vi "cRIO9159_DAQDMA.vi"() -> ()   [LabVIEW 2013]
uses:
  datatypes/statesdaq.ctl
  <vilib>/rvi/Emulation/niFpgaSctlEmulationGetInTimedLoop.vi
  <vilib>/rvi/Emulation/niFpgaEmulationReportErrorSimple.vi
  <vilib>/rvi/Emulation/niFpgaGetClockAttributes.vi
  <vilib>/rvi/eio/common/nirviEmuTemplatePropertyGet_noerrors.vi
  <vilib>/rvi/eio/common/nirviEmuTemplateMethod_errors.vi
  <vilib>/rvi/Emulation/niFpgaCriticalErrorInLSC.vi
  <vilib>/rvi/interface/RandomDataEmulation/nirviRandomDataFPGAFIFO.vi
  <vilib>/rvi/interface/RandomDataEmulation/niFpgaRandomDataHandleErrors.vi
  <vilib>/eio/EIOPropertyNode/EIOPropertyNode.xnode
  <vilib>/eio/EIOMethodNode/EIOMethodNode.xnode
  <vilib>/eio/EIONode/EIONode.xnode
  <vilib>/rvi/DataTransferAndStorage/Container/XNode/niFpgaContainer.xnode
  <vilib>/rvi/interface/RandomDataEmulation/nirviRandomDataFpgaReadWriteTemplate.vi
  <vilib>/rvi/eio/common/nirviEmuTemplatePropertyGet_errors.vi
  <vilib>/rvi/eio/common/nirviEmuTemplatePropertySet_errors.vi
  <vilib>/rvi/eio/common/nirviEmuTemplatePropertySet_noerrors.vi
panel:
  in  "Loop(uSec)":u32=1000 caption="Count(uSec)"
  in  "Tab Control":T1(tab)=enum."Mandatory Resources"
  out "Platform":enum8{"FlexRIO", "cRIO", "RSeries"}(ring)=enum."cRIO"
  out "FPGAVIversion":u8[](array[numeric])=[1, 1]
  out "InitDone":bool
  out "Fref":u32=1000
  out "DevQualityStatus":u8
  out "DevTemp":i16=-9378
  out "DevProfile":u8
  in  "DAQStartStop":bool
  in  "DebugMode":bool
  out "InsertedIOModulesID":u16[](array[numeric])
  out "cRIOModulesOK":bool
  out "DMATtoHOSTBlockNWords":u16[](array[numeric])=[128]
  out "DMATtoHOSTNCh":u16[](array[numeric])=[2]
  out "DMATtoHOSTFrameType":u8[](array[numeric])
  out "DMATtoHOSTSampleSize":u8[](array[numeric])=[4]
  out "DMATtoHOSTOverflows":u16
  in  "DMATtoHOSTSamplingRate0":u16=1
  in  "DMATtoHOSTEnable0":bool
  out "SGFref0":u32=10000
  in  "AOEnable2":bool
  in  "AOEnable1":bool
  out "SGNo":u8=1
  in  "AO0":i32
  in  "AO1":i32
  in  "AOEnable0":bool
  in  "SGFreq0":u32=100000
  in  "SGAmp0":u16
  in  "SGPhase0":u32
  in  "SGSignalType0":u8
  in  "SGUpdateRate0":u32=1
  in  "AO2":i32
  out "AI1":i32
  out "AI0":i32
  out "AI2":i32
  out "auxAI0":i32
  in  "auxAO0":i32
  out "DI0":bool
  out "DI1":bool
  in  "DO0":bool
  in  "DO1":bool
  out "auxDI0":bool
  in  "auxDO0":bool
  in  "DO2":bool
  out "DI2":bool
  out "state":T2=enum."acquisition"
  # "fref should be greater then (1/N*4us)"
  # "Analog Input"
  # "Aux Analog Input"
  # "Analog Output"
  # "Aux Analog Output"
  # "Signal Generator"
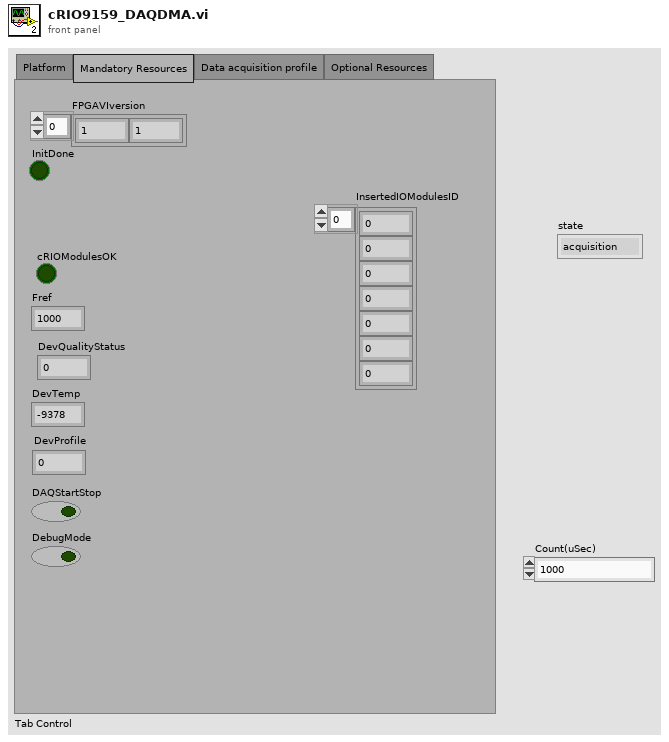
[diagram p1: front panel]
types:
  T1 = enum32{"Platform", "Mandatory Resources", "Data acquisition profile", "Optional Resources"}
  T2 = typedef "statesdaq.ctl" = enum16{"init", "waitingtrigger", "acquisition", "error"}
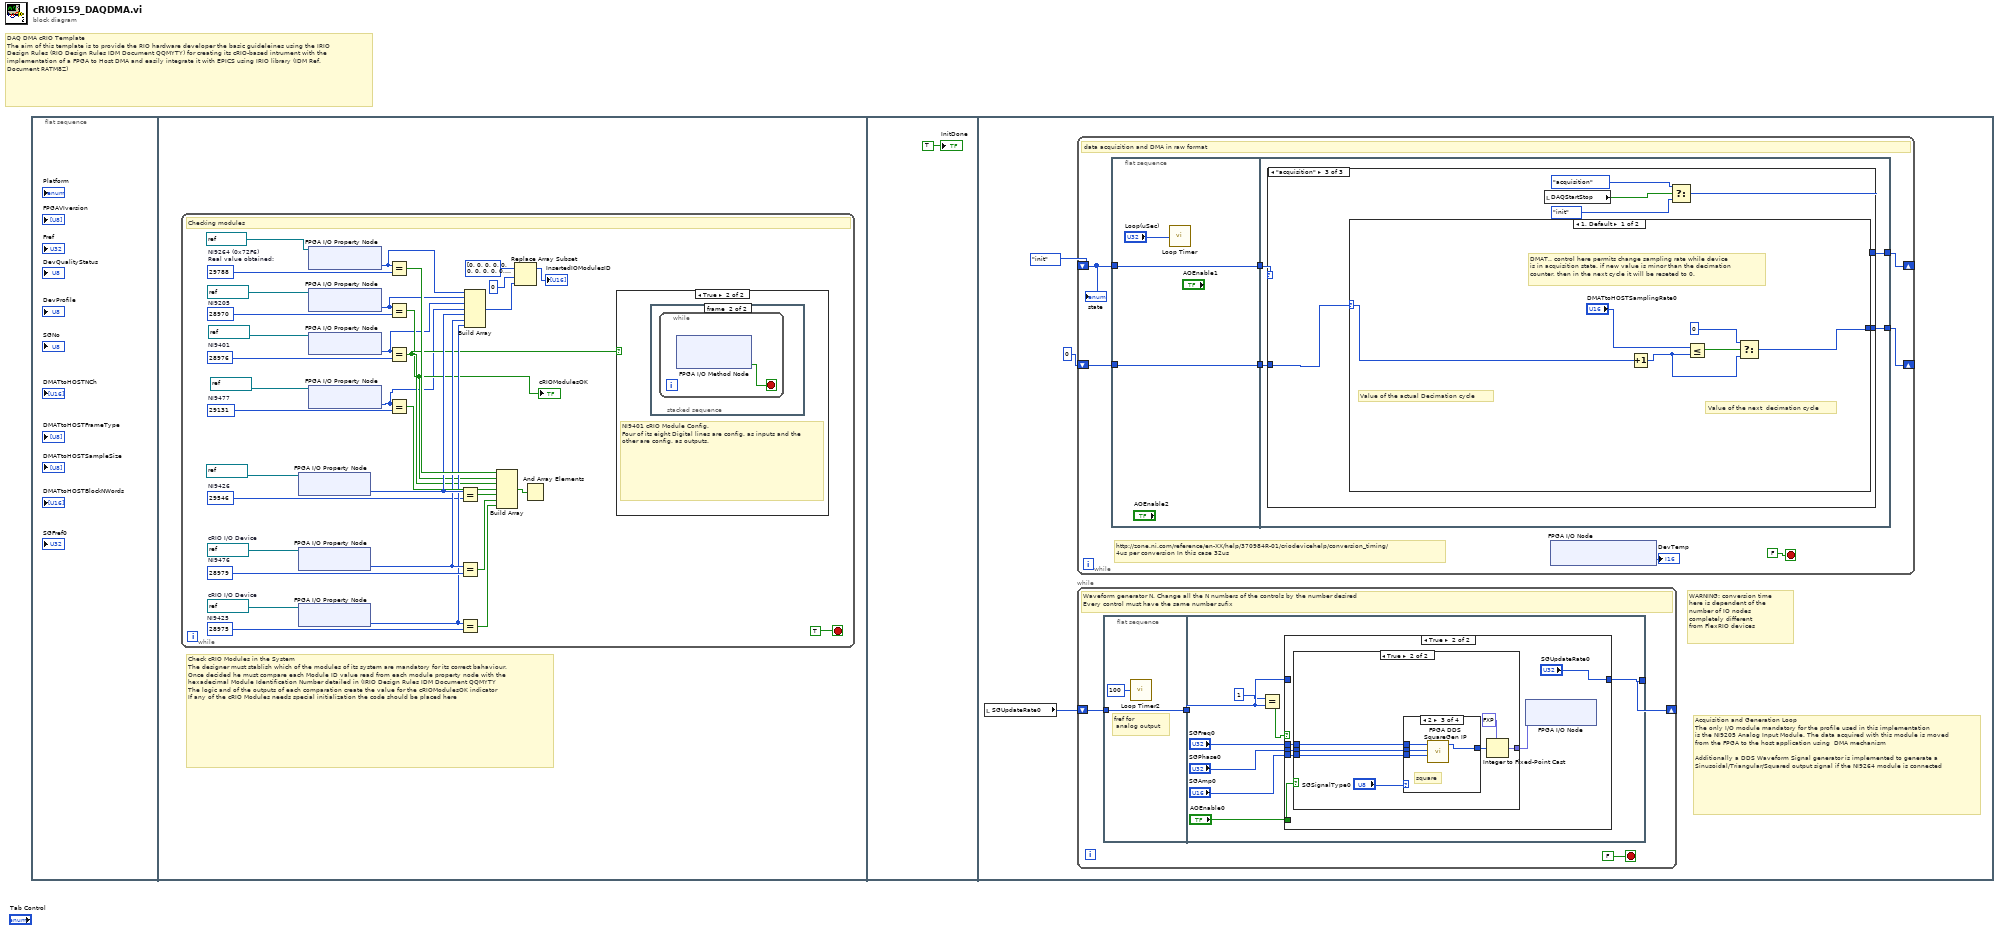
[diagram p0: block diagram]
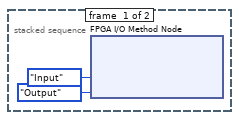
[diagram p3: hidden frame]
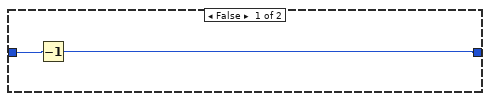
[diagram p4: hidden frame]
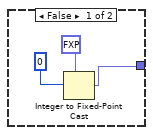
[diagram p5: hidden frame]
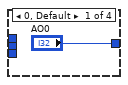
[diagram p6: hidden frame]
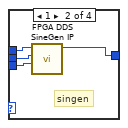
[diagram p7: hidden frame]
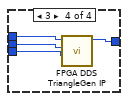
[diagram p8: hidden frame]
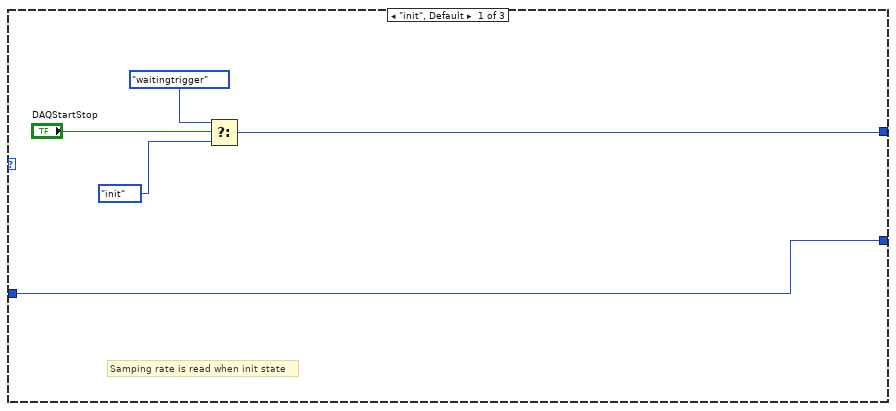
[diagram p9: hidden frame]
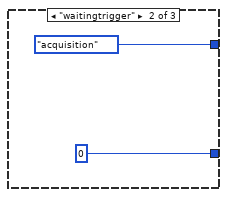
[diagram p10: hidden frame]
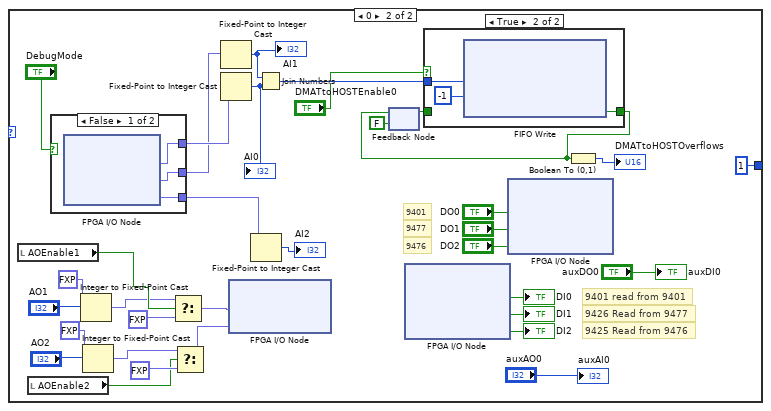
[diagram p11: hidden frame]
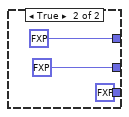
[diagram p13: hidden frame]
diagram:
  # "DAQ DMA cRIO Template\nThe aim of this template is to provide the RIO hardware developer the basic guideleines using the IRIO Design Rules (RIO Design Rules IDM Document QQMYTY) for creating its cRIO-based intrument with the implementation of a FPGA to Host DMA and easily integrate it with EPICS using IRIO library (IDM Ref. Document RATM8Z)"
  n1 = flat-sequence {
    frame #0 {
    }
    frame #1 {
      # "Check cRIO Modules in the System\nThe designer must stablish which of the modules of its system are mandatory for its correct bahaviour. \nOnce decided he must compare each Module ID value read from each module property node with the hexadecimal Module Identification Number detailed in (IRIO Design Rules IDM Document QQMYTY\nThe logic and of the outputs of each comparation create the value for the cRIOModulesOK indicator\nIf any of the cRIO Modules needs special initialization the code should be placed here"
      n2 = while {
        stop <- TRUE stop-if-true
        w13 = u16 28975  # NI9425
        w14 = u16 29546  # NI9426
        w7 = u16 29131  # NI9477
        w16 = u16 28976  # NI9401
        w8 = u16 28970  # NI9205
        w15 = u16 29788  # NI9264 (0x72F6)  Real value obtained:
        w18 = refnum<k21> "Mod7"  # cRIO I/O Device
        w19 = refnum<k21> "Mod6"  # cRIO I/O Device
        w28 = u16 28979  # NI9476
        # "Checking modules"
        n3 = xnode "FPGA I/O Property Node"("FPGA I/O In"=refnum<k21> "Mod5") -> ("Module ID"=w24:u16)  [unwired: 1 out]
        n4 = xnode "FPGA I/O Property Node"("FPGA I/O In"=w19) -> ("Module ID"=w23:u16)  [unwired: 1 out]
        n5 = xnode "FPGA I/O Property Node"("FPGA I/O In"=w18) -> ("Module ID"=w22:u16)  [unwired: 1 out]
        n6 = xnode "FPGA I/O Property Node"("FPGA I/O In"=refnum<k21> "Mod1") -> ("Module ID"=w4:u16)  [unwired: 1 out]
        n7 = xnode "FPGA I/O Property Node"("FPGA I/O In"=refnum<k21> "Mod2") -> ("Module ID"=w3:u16)  [unwired: 1 out]
        n8 = xnode "FPGA I/O Property Node"("FPGA I/O In"=refnum<k21> "Mod3") -> ("Module ID"=w2:u16)  [unwired: 1 out]
        n9 = xnode "FPGA I/O Property Node"("FPGA I/O In"=refnum<k21> "Mod4") -> ("Module ID"=w1:u16)  [unwired: 1 out]
        n10 = Equal?(x=w4, y=w15) -> (x = y?=w34:bool)
        n11 = Equal?(x=w3, y=w8) -> (x = y?=w5:bool)
        "cRIOModulesOK" <- w5
        n12 = Equal?(x=w2, y=w16) -> (x = y?=w6:bool)
        n13 = Equal?(x=w1, y=w7) -> (x = y?=w33:bool)
        n14 = Equal?(x=w24, y=w14) -> (x = y?=w32:bool)
        n15 = Equal?(x=w23, y=w28) -> (x = y?=w31:bool)
        n16 = Equal?(x=w22, y=w13) -> (x = y?=w30:bool)
        n17 = Build Array(w4, w3, w2, w1, w24, w23, w22) -> (w21:u16[])
        n18 = Build Array(w34, w5, w6, w33, w32, w31, w30) -> (w29:bool[])
        n19 = Replace Array Subset(array=u16[] [0, 0, 0, 0, 0, 0, 0, 0, 0, 0, 0, 0, 0, 0, 0, 0] ("InsertedIOModulesID"), new element=w21, index=0) -> (→"InsertedIOModulesID":u16[])
        n20 = And Array Elements(Boolean array=w29) -> ()  [unwired: 1 out]
        n21 = case shown="True" w6 {
          frame False {
          }
          frame True {
            # "NI9401 cRIO Module Config.\nFour of its eight Digital lines are config. as inputs and the other are config. as outputs."
            n22 = stacked-sequence {
              frame #0 {
                n23 = xnode "FPGA I/O Method Node"("DIO 7:4"=enum8{"No Change", "Input", "Output"}."Input", "DIO 3:0"=enum8{"No Change", "Input", "Output"}."Output") -> ()  [unwired: 1 in, 1 out]
              }
              frame #1 {
                n24 = while {
                  stop <- w37 stop-if-true
                  n25 = xnode "FPGA I/O Method Node"() -> ("Ready"=w37:bool)  [unwired: 1 in, 1 out]
                }
              }
            }
          }
        }
      }
    }
    frame #2 {
      "InitDone" <- TRUE ("InitDone")
    }
    frame #3 {
      # "Acquisition and Generation Loop\nThe only I/O module mandatory for the profile used in this implementation \nis the NI9205 Analog Input Module. The data acquired with this module is moved from the FPGA to the host application using  DMA mechanism\n\nAdditionally a DDS Waveform Signal generator is implemented to generate a Sinusoidal/Triangular/Squared output signal if the NI9264 module is connected"
      # "WARNING: conversion time \nhere is dependent of the \nnumber of IO nodes\ncompletely different \nfrom FlexRIO devices"
      n26 = local read "SGUpdateRate0"() -> (w39:u32)
      n27 = while {
        shift-right: [w42] -> _
        shift-left: w39 -> [w43]
        stop <- FALSE stop-if-true
        # "Waveform generator N. Change all the N numbers of the controls by the number desired\nEvery control must have the same number sufix"
        n28 = flat-sequence {
          tunnel: [w46] -> w44
          tunnel: w43 -> [w46]
          tunnel: w44 -> [w50]
          tunnel: [w49] -> w42
          frame #0 {
            # "fref for\n analog output"
            n29 = call "Loop Timer2"("Count(uSec)"=u32 100) -> ()  [unwired: 1 out]
          }
          frame #1 {
            n30 = Equal?(x=u32 1, y=w50) -> (x = y?=w51:bool)
            n31 = case shown="True" w51 {
              tunnel: "SGFreq0" -> [_ w63]
              tunnel: "SGPhase0" -> [_ w62]
              tunnel: "SGAmp0" -> [_ w61]
              tunnel: "AOEnable0" -> [_ w60]
              tunnel: w50 -> [w57 _]
              tunnel: [w56 "SGUpdateRate0"] -> w49
              frame False {
                n32 = Decrement(x=w57) -> (x-1=w56:u32)
              }
              frame True {
                n33 = case shown="True" w60 {
                  tunnel: w63 -> [_ w73]
                  tunnel: w62 -> [_ w72]
                  tunnel: w61 -> [_ w71]
                  tunnel: [w64 w68] -> w59
                  frame False {
                    n34 = Integer to Fixed-Point Cast(fixed-point type=fxp<+/-,20,5> 0.0 ("f"), integer=i16 0) -> (fixed-point=w64:fxp<+/-,20,5>)
                  }
                  frame True {
                    n35 = case shown="2" "SGSignalType0" {
                      tunnel: w73 -> [_ w78 w82 w86]
                      tunnel: w72 -> [_ w77 w81 w85]
                      tunnel: w71 -> [_ w76 w80 w84]
                      tunnel: ["AO0" w75 w79 w83] -> w69
                      frame 0, Default {
                      }
                      frame 1 {
                        # "singen"
                        n36 = call "FPGA DDS SineGen IP.vi"("Signal Amplitude (x 2^15)"=w76, "Phase Shift"=w77, "Accumulator Increment"=w78) -> ("Signal Value"=w75:i16)  [unwired: 7 in, 1 out]
                      }
                      frame 2 {
                        # "square"
                        n37 = call "FPGA DDS SquareGen IP.vi"("Signal Amplitude (x 2^15)"=w80, "Phase Shift"=w81, "Accumulator Increment"=w82) -> ("Signal Value"=w79:i16)  [unwired: 7 in, 1 out]
                      }
                      frame 3 {
                        n38 = call "FPGA DDS TriangleGen IP.vi"("Signal Amplitude (x 2^15)"=w84, "Phase Shift"=w85, "Accumulator Increment"=w86) -> ("Signal Value"=w83:i16)  [unwired: 7 in, 1 out]
                      }
                    }
                    n39 = Integer to Fixed-Point Cast(fixed-point type=fxp<+/-,20,5> 0.0 ("f"), integer=w69) -> (fixed-point=w68:fxp<+/-,20,5>)
                  }
                }
                n40 = xnode "FPGA I/O Node"("Mod1/AO0"=w59) -> ()  [unwired: 1 in, 1 out]
              }
            }
          }
        }
      }
      n41 = while {
        shift-right: [w91] -> _
        shift-left: statesdaq."init" -> [w92]
        shift-right: [w89] -> _
        shift-left: u16 0 -> [w87]
        stop <- FALSE stop-if-true
        # "http://zone.ni.com/reference/en-XX/help/370984R-01/criodevicehelp/conversion_timing/\n4us per conversion In this case 32us"
        # "data acquisition and DMA in raw format"
        n42 = flat-sequence {
          tunnel: [w96] -> w93
          tunnel: w92 -> [w96]
          tunnel: [w95] -> w88
          tunnel: w87 -> [w95]
          tunnel: w93 -> [w101]
          tunnel: [w100] -> w91
          tunnel: [w99] -> w89
          tunnel: w88 -> [w98]
          frame #0 {
            n43 = call "Loop Timer"("Count(uSec)"="Loop(uSec)") -> ()  [unwired: 1 out]
          }
          frame #1 {
            n44 = case shown="\"acquisition\"" w101 {
              tunnel: [w103 statesdaq."acquisition" w111] -> w100
              tunnel: [w102 i16 0 w110] -> w99
              tunnel: w98 -> [w102 _ w109]
              frame "init", Default {
                # "Samping rate is read when init state"
                n45 = Select(t=statesdaq."waitingtrigger", s="DAQStartStop", f=statesdaq."init") -> (s? t:f=w103:T2)
              }
              frame "waitingtrigger" {
              }
              frame "acquisition" {
                n46 = case shown="1, Default" w109 {
                  selector: w109 -> [w120 _]
                  tunnel: [w115 u16 1] -> w110
                  frame 1, Default {
                    # "DMAT.. control here permits change sampling rate while device\nis in acquisition state. if new value is minor than the decimation \ncounter, then in the next cycle it will be reseted to 0."
                    # "Value of the next  decimation cycle"
                    # "Value of the actual Decimation cycle"
                    n47 = Increment(x=w120) -> (x+1=w116:u16)
                    n48 = Less Or Equal?(x="DMATtoHOSTSamplingRate0", y=w116) -> (x <= y?=w118:bool)
                    n49 = Select(t=u16 0, s=w118, f=w116) -> (s? t:f=w115:u16)
                  }
                  frame 0 {
                    # "9425 Read from 9476"
                    # "9426 Read from 9477"
                    # "9401 read from 9401"
                    # "9476"
                    # "9477"
                    # "9401"
                    n50 = local read "AOEnable1"() -> (w146:bool)
                    n51 = local read "AOEnable2"() -> (w136:bool)
                    n52 = case shown="False" "DebugMode" {
                      tunnel: [w161 fxp<+/-,26,5> 5.0 ("fixed-point")] -> w150
                      tunnel: [w160 fxp<+/-,26,5> -5.0 ("fixed-point")] -> w149
                      tunnel: [w159 fxp<+/-,26,5> 2.0 ("Mod3/AI0")] -> w133
                      frame False {
                        n53 = xnode "FPGA I/O Node"() -> ("Mod2/AI0"=w161:fxp<+/-,26,5>, "Mod2/AI1"=w160:fxp<+/-,26,5>, "Mod2/AI2"=w159:fxp<+/-,26,5>)  [unwired: 3 in, 3 out]
                      }
                      frame True {
                      }
                    }
                    n54 = Integer to Fixed-Point Cast(fixed-point type=fxp<+/-,20,5> 0.0, integer="AO1") -> (fixed-point=w144:fxp<+/-,20,5>)
                    n55 = Integer to Fixed-Point Cast(fixed-point type=fxp<+/-,20,5> 0.0, integer="AO2") -> (fixed-point=w138:fxp<+/-,20,5>)
                    n56 = Select(t=w144, s=w146, f=fxp<+/-,20,5> 0.0) -> (s? t:f=w142:fxp<+/-,20,5>)
                    n57 = Select(t=w138, s=w136, f=fxp<+/-,20,5> 0.0) -> (s? t:f=w135:fxp<+/-,20,5>)
                    n58 = Fixed-Point to Integer Cast(1:w149) -> (0:w154:i32)
                    "AI1" <- w154
                    n59 = Fixed-Point to Integer Cast(1:w150) -> (0:w153:i32)
                    "AI0" <- w153
                    n60 = xnode "FPGA I/O Node"("Mod1/AO1"=w142, "Mod1/AO2"=w135) -> ()  [unwired: 2 in, 2 out]
                    n61 = Fixed-Point to Integer Cast(1:w133) -> (0:→"AI2":i32)
                    n62 = Join Numbers(hi=w154, lo=w153) -> ((hi.lo)=w148:u64)
                    n63 = feedback #1(FALSE ("Timed Out?")) -> (w131:bool)
                    n64 = xnode "FPGA I/O Node"() -> ("Mod3/DIO4"=→"DI0":bool, "Mod5/DI0"=→"DI1":bool, "Mod7/DI0"=→"DI2":bool)  [unwired: 4 in, 4 out]
                    n65 = case shown="True" "DMATtoHOSTEnable0" {
                      tunnel: w148 -> [_ w157]
                      tunnel: [w155 w156] -> w130
                      tunnel: w131 -> [w155 _]
                      frame False {
                      }
                      frame True {
                        n66 = xnode ("FIFO Write")("Element"=w157, "Timeout"=-1) -> ("Timed Out?"=w156:bool)  [unwired: 1 in, 1 out]
                      }
                    }
                    n67 = feedback-in #1(w130) -> ()
                    n68 = xnode "FPGA I/O Node"("Mod3/DIO0"="DO0", "Mod4/DO0"="DO1", "Mod6/DO0"="DO2") -> ()  [unwired: 4 in, 4 out]
                    n69 = Boolean To (0,1)(Boolean=w130) -> (0, 1=→"DMATtoHOSTOverflows":i16)
                    "auxAI0" <- "auxAO0"
                    "auxDI0" <- "auxDO0"
                  }
                }
                n70 = local read "DAQStartStop"() -> (w114:bool)
                n71 = Select(t=statesdaq."acquisition", s=w114, f=statesdaq."init") -> (s? t:f=w111:T2)
              }
            }
          }
        }
        n72 = xnode "FPGA I/O Node"() -> ("Chassis Temperature"=→"DevTemp":i16)  [unwired: 1 in, 1 out]
        "state" <- w92
      }
    }
  }
